vi "Destroy UI Display.vi"(8 "error in (no error)":errorcluster, 11 "References in":T1) -> (0 "error out":errorcluster, 3 "References out":T1)   [LabVIEW 2021, in "Build Script Common.lvlib"]
uses:
  Build Script Common.lvlib
  Typedef/References.ctl
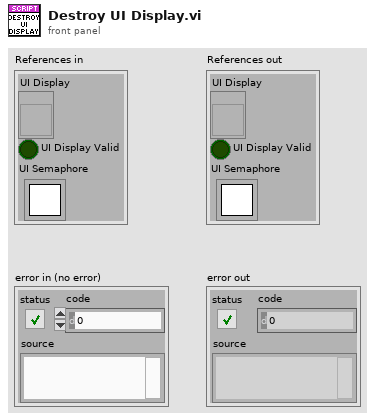
[diagram p1: front panel]
types:
  T1 = typedef "Build Script Common.lvlib/References.ctl" = cluster{"UI Display":refnum<vi>, "UI Display Valid":bool, "UI Semaphore":T2}
  T2 = typedef "Semaphore RefNum" = refnum<k1>
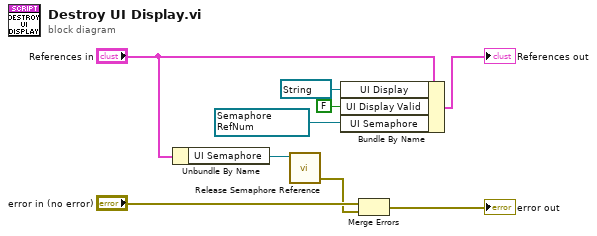
[diagram p0: block diagram]
diagram:
  w4 = T2 refnum items=["semaphore"] ("UI Semaphore")
  n1 = Unbundle By Name("References in") -> ("UI Semaphore"=w6:T2)
  n2 = call <vilib>:"Release Semaphore Reference.vi"("semaphore"=w6) -> ("error out"=w2:errorcluster)  [unwired: 9 in, 1 out]
  n3 = Bundle By Name(cluster="References in", "UI Display"=refnum<vi> refnum, "UI Display Valid"=FALSE, "UI Semaphore"=w4) -> (→"References out":T1)
  n4 = Merge Errors("error in (no error)", w2) -> (→"error out":errorcluster)
